vi "cameraGlobal.vi"() -> ()   [LabVIEW 2013]
panel:
  in  "Slit Width / Number of Lines":sgl=200.0
  in  "LinesToReadout":sgl=2048.0 min=1 max=2048 step=1
  out "Frame Interval (sec)":sgl=0.100005634
  out "Line Interval Set (sec)":sgl=4.4289474e-05 format="%#_9p"
  in  "Readout Direction":sgl(ring)=1.0 items=["Forward"=1, "Backward"=2]
  in  "Trigger Mode":sgl(ring)=1.0 items=["Normal"=1, "Start "=6]
  in  "Trigger Source":sgl(ring)=2.0 items=["Internal"=1, "External"=2]
  out "Full Frame Exp Time Set (sec)":sgl=0.10000638
  in  "Full Frame Exposure Time (sec)":dbl=0.1
  out "Slit Scanning Expos Time Set (sec)":sgl=0.008857895
  in  "Slit Scanning Exposure Time (sec)":dbl=0.008857395925597875 format="%#_6p"
  in  "Line Interval (sec)":sgl=4.428698e-05 format="%#_6p"
  in  "Camera Readout Mode":u16(ring)=12 items=["Full Frame"=1, "Slit Scanning"=12]
  out "Camera Handle":u32
  out "Camera Serial":string="S/N: 750964"
  out "Camera Version":string="2.50.A"
  out "Camera Model":string="C11440-22C"
  # "Sensor Mode \n1: full chip\n12: progressive,lightsheet"
  # "Trigger Source, \n1: Internal \n2: External"
  # "Trigger Mode, \n1: Normal, \n6: Start on Trigger"
  # "Readout Direction \n1: Top to Bottom, \n2: Bottom to Top"
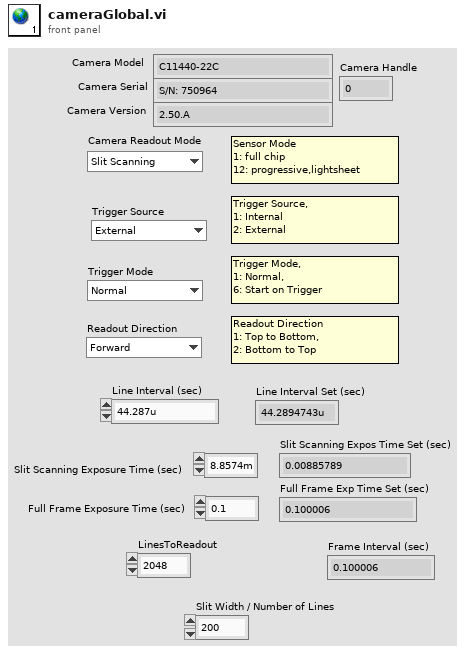
[diagram p1: front panel]
diagram:
